vi "BRig_Host_dataRunState_dataPlot_unknown.vi"() -> (2 "output_idx_dataPlot_unknown":i32)   [LabVIEW 2014]
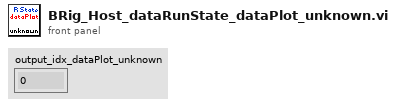
[diagram p1: front panel]
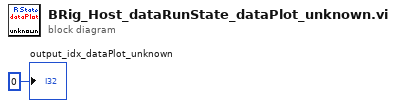
[diagram p0: block diagram]
diagram:
  "output_idx_dataPlot_unknown" <- 0 ("output_idx_dataTS")
